vi "MacroInterpreter_MD.vi"() -> ()   [LabVIEW 2012]
uses:
  SubVIs/Timer_MacroInterpreter_Commands.ctl
  GFG/GFG library.lvlib
panel:
  out "number 3":dbl
  out "number 2":dbl
  out "number":dbl
  in  "stop":bool
  out "Error Out":errorcluster
  in  "Error In":errorcluster
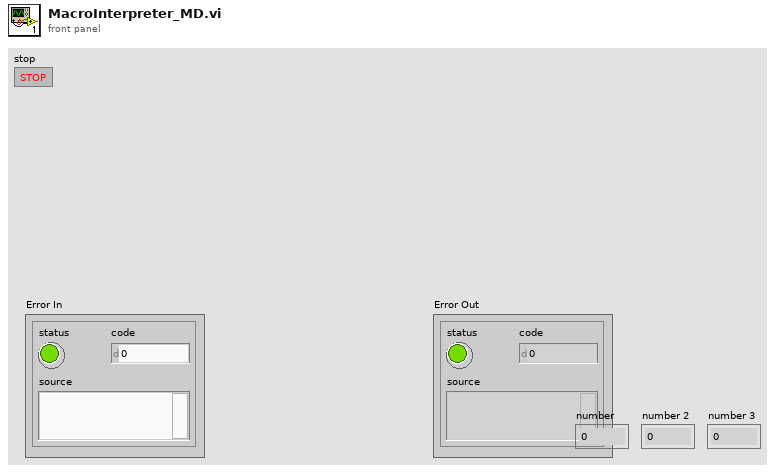
[diagram p1: front panel]
types:
  T1 = typedef "Timer_MacroInterpreter_Commands.ctl" = enum16{"Start", "Pause", "Run"}
  T2 = cluster{"moveXabs":dbl, "moveYabs":dbl, "moveZabs":dbl}
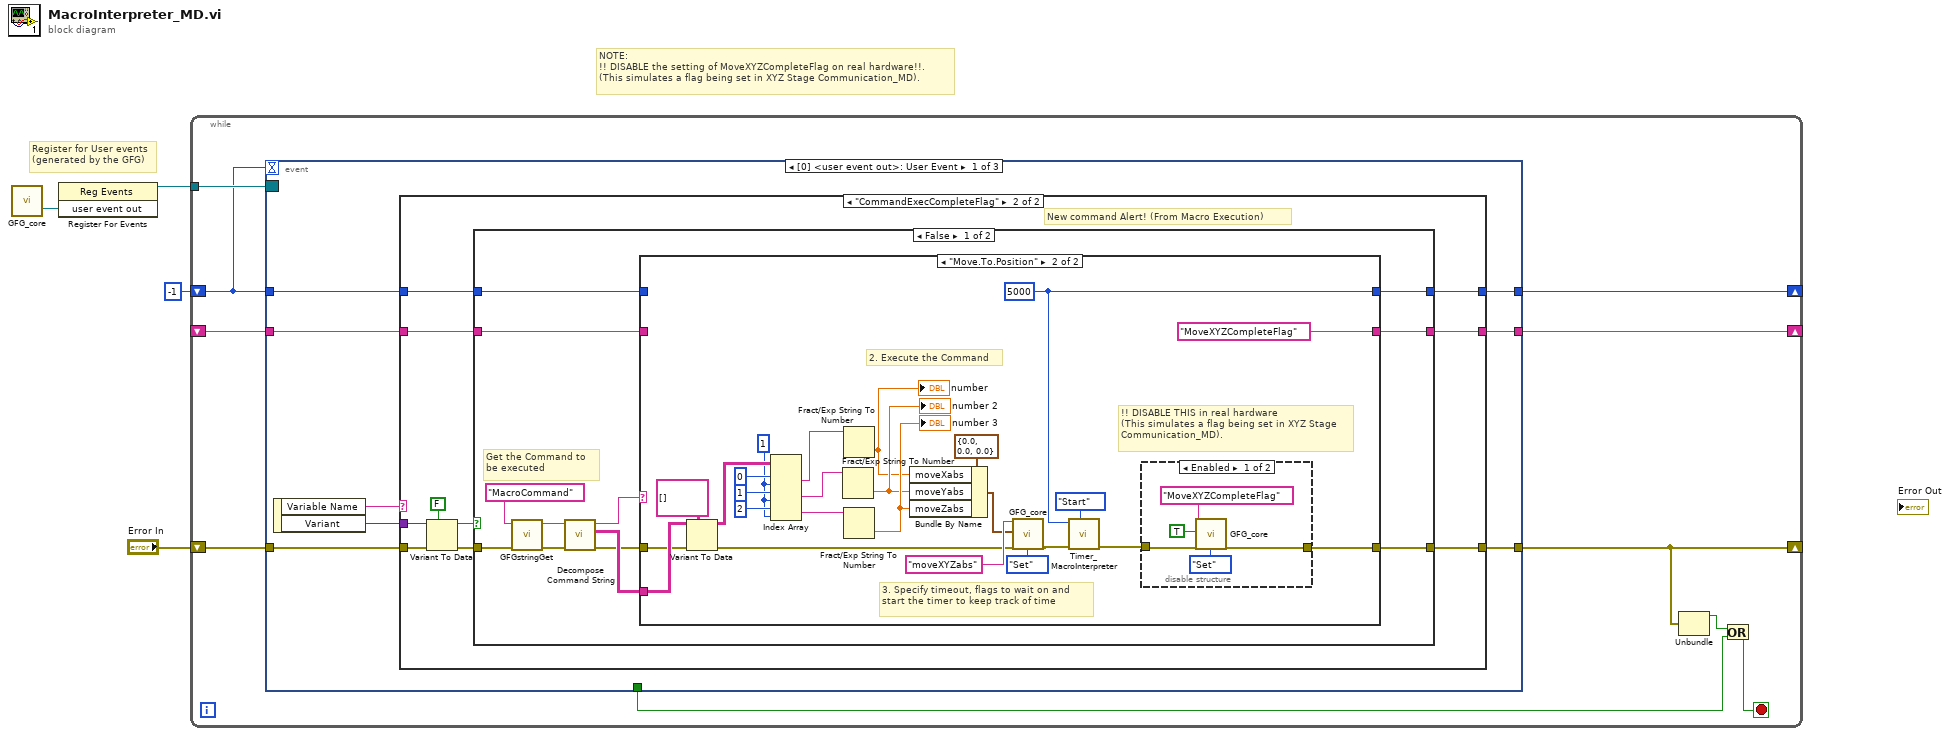
[diagram p0: block diagram]
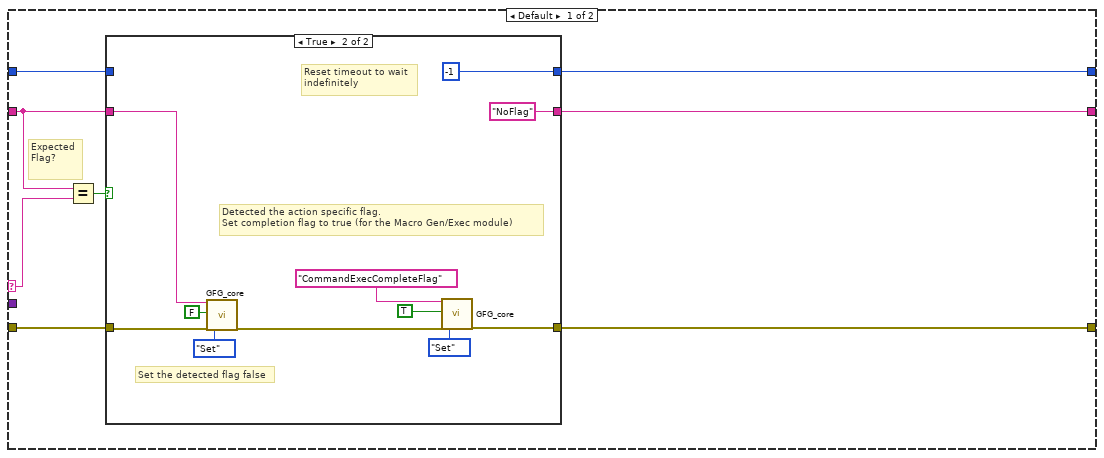
[diagram p2: hidden frame]
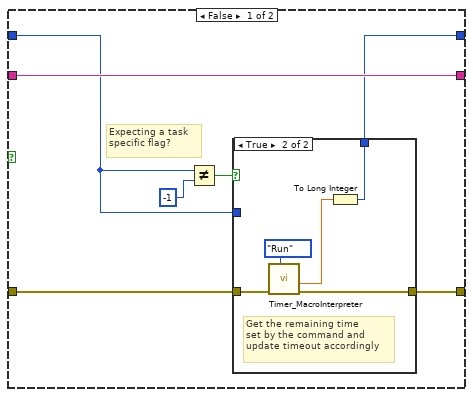
[diagram p3: hidden frame]
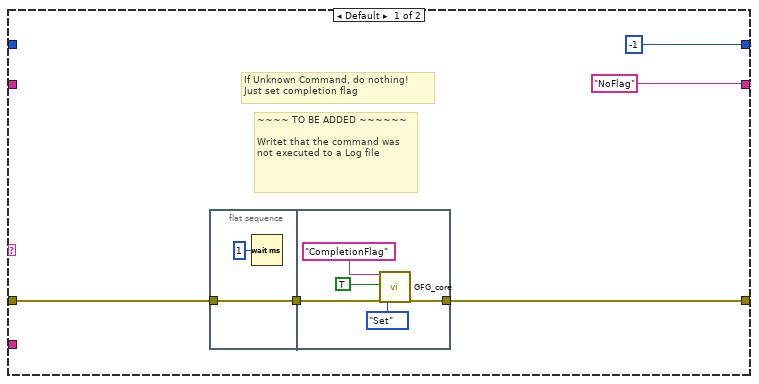
[diagram p5: hidden frame]
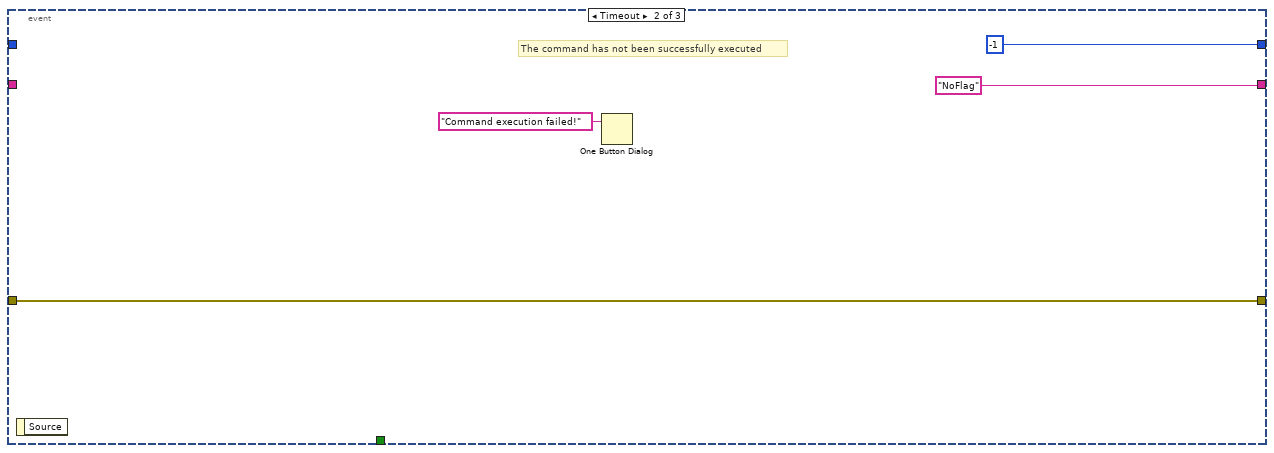
[diagram p8: hidden frame]
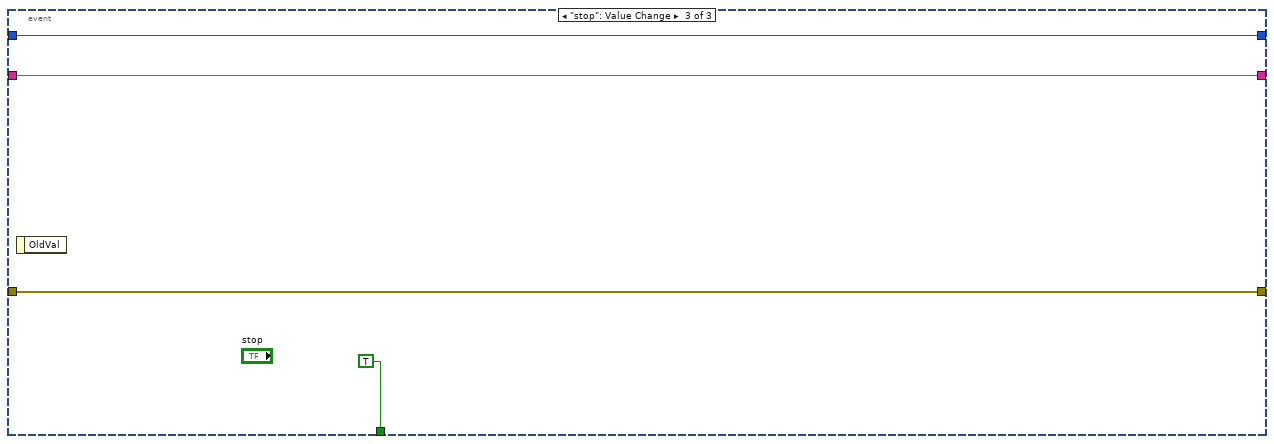
[diagram p9: hidden frame]
diagram:
  # "NOTE:\n!! DISABLE the setting of MoveXYZCompleteFlag on real hardware!!.\n(This simulates a flag being set in XYZ Stage Communication_MD)."
  # "Register for User events\n(generated by the GFG)"
  n1 = call "GFG_core.vi"() -> ("user event out"=w4:refnum<user-event>)  [unwired: 13 in, 6 out]
  n2 = register-events(w4) -> (reference out=w3:refnum<event-registration>)  [unwired: 2 in, 1 out]
  n3 = while {
    tunnel: w3 -> [w14]
    shift-right: [w12] -> _
    shift-left: _ -> [w11]
    shift-right: [w10] -> _
    shift-left: -1 -> [w9]
    shift-right: [w8] -> _
    shift-left: "Error In" -> [w13]
    stop <- w5 stop-if-true
    n4 = event shown="[0] <user event out>: User Event" {
      selector: w14 -> [_ _ _]
      dyn-events: _ -> [_ _ _]
      timeout: w9 -> [_ _ _]
      tunnel: w13 -> [w21 w123 w126]
      tunnel: [_ _ TRUE] -> w6
      tunnel: [w19 "NoFlag" ("Variable Name in") w128] -> w12
      tunnel: w11 -> [w16 _ w128]
      tunnel: [w18 -1 w127] -> w10
      tunnel: w9 -> [w17 _ w127]
      tunnel: [w15 w123 w126] -> w8
      event User Event {
        n5 = event-data() -> ("Variable Name"=w22:string, "Variant"=w20:variant)  [unwired: 1 in]
        n6 = case shown="\"CommandExecCompleteFlag\"" w22 {
          selector: w22 -> [w30 _]
          tunnel: w21 -> [w23 w63]
          tunnel: w20 -> [_ w64]
          tunnel: [w26 w60] -> w19
          tunnel: [w28 w59] -> w18
          tunnel: w17 -> [w29 w58]
          tunnel: w16 -> [w27 w57]
          tunnel: [w25 w56] -> w15
          frame Default {
            # "Expected Flag?"
            n7 = Equal?(x=w27, y=w30) -> (x = y?=w24:bool)
            n8 = case shown="True" w24 {
              tunnel: w29 -> [w31 _]
              tunnel: [w32 -1] -> w28
              tunnel: [w37 "NoFlag" ("Variable Name in")] -> w26
              tunnel: w27 -> [w37 w46]
              tunnel: w23 -> [w34 w47]
              tunnel: [w33 w50] -> w25
              frame False {
                # "Expecting a task specific flag?"
                n9 = Not Equal?(x=w31, y=-1) -> (x != y?=w35:bool)
                n10 = case shown="True" w35 {
                  tunnel: w34 -> [w38 w43]
                  tunnel: [w38 w41] -> w33
                  tunnel: [w39 w40] -> w32
                  tunnel: w31 -> [w39 _]
                  frame False {
                    # "Wait indefinitely\n(timeout = -1)"
                  }
                  frame True {
                    # "Get the remaining time\nset by the command and\nupdate timeout accordingly"
                    n11 = call "Timer_MacroInterpreter.vi"("Timer Command"=Timer_MacroInterpreter_Commands."Run", "Error In"=w43) -> ("Error Out"=w41:errorcluster, "Remaining Time (ms)"=w42:dbl)  [unwired: 6 in, 2 out]
                    n12 = To Long Integer(number=w42) -> (32bit integer=w40:i32)
                  }
                }
              }
              frame True {
                # "Reset timeout to wait\nindefinitely"
                # "Set the detected flag false"
                # "Detected the action specific flag.\nSet completion flag to true (for the Macro Gen/Exec module)"
                n13 = call "GFG_core.vi"("Variable Name in"=w46, "Variant in"=FALSE, "error in (no error)"=w47, "Action"=enum16{"Init", "Set", "Get", "Clear"}."Set") -> ("error out"=w45:errorcluster)  [unwired: 9 in, 6 out]
                n14 = call "GFG_core.vi"("Variable Name in"="CommandExecCompleteFlag", "Variant in"=TRUE, "error in (no error)"=w45, "Action"=enum16{"Init", "Set", "Get", "Clear"}."Set") -> ("error out"=w50:errorcluster)  [unwired: 9 in, 6 out]
              }
            }
          }
          frame "CommandExecCompleteFlag" {
            # "New command Alert! (From Macro Execution)"
            n15 = Variant To Data(error in=w63, type=FALSE, Variant=w64) -> (data=w62:bool, error out=w61:errorcluster)
            n16 = case shown="False" w62 {
              tunnel: w61 -> [w71 w119]
              tunnel: [w70 w120] -> w60
              tunnel: [w69 w121] -> w59
              tunnel: w58 -> [w67 w121]
              tunnel: w57 -> [w68 w120]
              tunnel: [w66 w119] -> w56
              frame False {
                # "Get the Command to\nbe executed"
                n17 = call "GFGstringGet.vi"("Variable Name in"="MacroCommand" ("Source VI")) -> ("String"=w74:string)  [unwired: 10 in]
                n18 = call "Decompose Command String.vi"("Error In"=w71, "Command IN"=w74) -> ("Error Out"=w72:errorcluster, "ArgumentTable"=w73:string[][], "Action"=w76:string)  [unwired: 7 in]
                n19 = case shown="\"Move.To.Position\"" w76 {
                  tunnel: w73 -> [_ w96]
                  tunnel: w72 -> [w80 w91]
                  tunnel: ["NoFlag" ("Variable Name in") "MoveXYZCompleteFlag" ("Variable Name in")] -> w70
                  tunnel: [-1 w93] -> w69
                  tunnel: w68 -> [_ _]
                  tunnel: w67 -> [_ _]
                  tunnel: [w77 w89] -> w66
                  frame Default {
                    # "~~~~ TO BE ADDED ~~~~~~\n\nWritet that the command was not executed to a Log file"
                    # "If Unknown Command, do nothing!\nJust set completion flag"
                    n20 = flat-sequence {
                      tunnel: [w82] -> w81
                      tunnel: w80 -> [w82]
                      tunnel: w81 -> [w85]
                      tunnel: [w84] -> w77
                      frame #0 {
                        n21 = Wait (ms)(milliseconds to wait=u32 1) -> ()  [unwired: 1 out]
                      }
                      frame #1 {
                        n22 = call "GFG_core.vi"("Variable Name in"="CompletionFlag", "Variant in"=TRUE, "error in (no error)"=w85, "Action"=enum16{"Init", "Set", "Get", "Clear"}."Set") -> ("error out"=w84:errorcluster)  [unwired: 9 in, 6 out]
                      }
                    }
                  }
                  frame "Move.To.Position" {
                    w93 = 5000
                    w108 = 1 ("disabled index (col)")
                    # "!! DISABLE THIS in real hardware\n(This simulates a flag being set in XYZ Stage\nCommunication_MD)."
                    # "3. Specify timeout, flags to wait on and start the timer to keep track of time"
                    # "2. Execute the Command"
                    n23 = Variant To Data(error in=w91, type=string[][] [], Variant=w96) -> (data=w112:string[][], error out=w100:errorcluster)
                    n24 = Index Array(array=w112, index (row) #1=0 ("disabled index (row)"), index (col) #1=w108, index (row) #2=1 ("disabled index (row)"), index (col) #2=w108, index (row) #3=2 ("disabled index (row)"), index (col) #3=w108) -> (element #1=w107:string, element #2=w106:string, element #3=w105:string)
                    n25 = Fract/Exp String To Number(string=w106) -> (number=w98:dbl)  [unwired: 3 in, 1 out]
                    "number 2" <- w98
                    n26 = Fract/Exp String To Number(string=w107) -> (number=w97:dbl)  [unwired: 3 in, 1 out]
                    "number" <- w97
                    n27 = Fract/Exp String To Number(string=w105) -> (number=w99:dbl)  [unwired: 3 in, 1 out]
                    "number 3" <- w99
                    n28 = Bundle By Name(cluster=T2 {"moveXabs"=0.0, "moveYabs"=0.0, "moveZabs"=0.0} ("output cluster"), "moveXabs"=w97, "moveYabs"=w98, "moveZabs"=w99) -> (w101:T2)
                    n29 = call "GFG_core.vi"("Variable Name in"="moveXYZabs", "Variant in"=w101, "error in (no error)"=w100, "Action"=enum16{"Init", "Set", "Get"}."Set") -> ("error out"=w92:errorcluster)  [unwired: 9 in, 6 out]
                    n30 = call "Timer_MacroInterpreter.vi"("Timer Command"=Timer_MacroInterpreter_Commands."Start", "Error In"=w92, "Set Time (ms)"=w93) -> ("Error Out"=w90:errorcluster)  [unwired: 5 in, 3 out]
                    n31 = disable-structure shown="Enabled" {
                      disable-tunnel: w90 -> [w118 _]
                      disable-tunnel: [w117 _] -> w89
                      frame Enabled {
                        n32 = call "GFG_core.vi"("Variable Name in"="MoveXYZCompleteFlag", "Variant in"=TRUE, "error in (no error)"=w118, "Action"=enum16{"Init", "Set", "Get"}."Set") -> ("error out"=w117:errorcluster)  [unwired: 9 in, 6 out]
                      }
                      frame Disabled {
                      }
                    }
                  }
                }
              }
              frame True {
                # "UNexpected value!  (Expecting a FALSE for the \"CompletionFlag\").\n -- Do nothing --"
              }
            }
          }
        }
      }
      event Timeout {
        # "The command has not been successfully executed"
        n33 = event-data() -> ()  [unwired: 1 in, 1 out]
        n34 = One Button Dialog(message="Command execution failed!") -> ()  [unwired: 1 in, 1 out]
      }
      event "stop": Value Change {
        n35 = event-data() -> ()  [unwired: 1 in, 1 out]
      }
    }
    n36 = Unbundle(w8) -> ("status"=w7:bool)  [unwired: 2 out]
    n37 = Or(x=w7, y=w6) -> (x .or. y?=w5:bool)
  }
